vi "Calculate Sample Rate.vi"(0 "data clock rate":dbl=120000000.0 format="%#.3pS/s", 5 "sample rate":dbl=10000000.0 format="%#.3pS/s") -> (4 "decimation sample rate":fxp<+,48,1>, 6 "coerced sample rate":dbl=10000000.0 min=1.0 max=250000000.0 format="%#.3pS/s")   [LabVIEW 2018]
doc: "Calculates the sample rate value to write to the DSP blocks of the device for a requested sample rate, in samples per second."
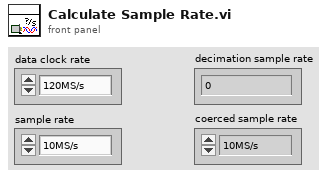
[diagram p1: front panel]
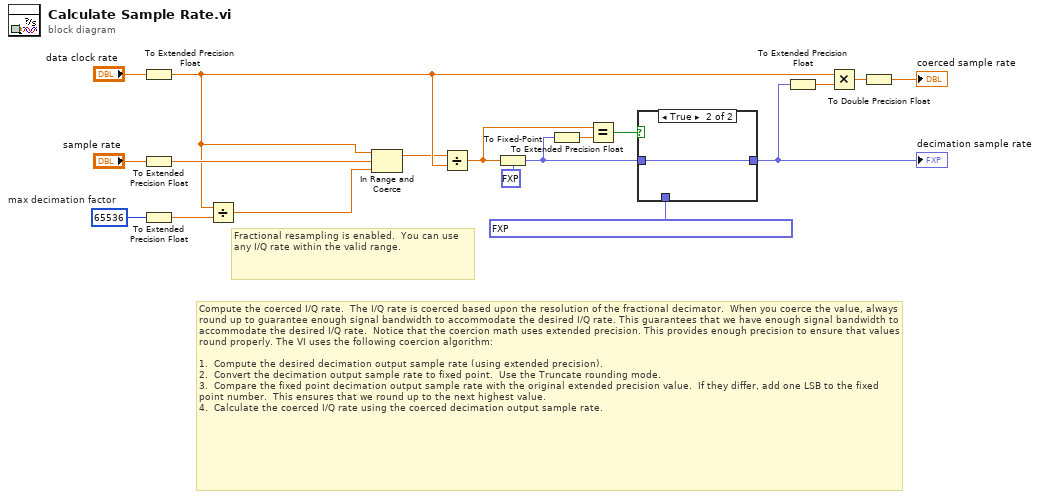
[diagram p0: block diagram]
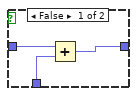
[diagram p2: hidden frame]
diagram:
  w3 = u32 65536  # max decimation factor
  # "Fractional resampling is enabled.  You can use any I/Q rate within the valid range."
  # "Compute the coerced I/Q rate.  The I/Q rate is coerced based upon the resolution of the fractional decimator.  When you coerce the value, always round up to guarantee enough signal bandwidth to accommodate the desired I/Q rate. This guarantees that we have enough signal bandwidth to accommodate the desired I/Q rate.  Notice that the coercion math uses extended precision. This provides enough precision to ensure that values round properly. The VI uses the following coercion algorithm:\n\n1.  Compute the desired decimation output sample rate (using extended precision).\n2.  Convert the decimation output sample rate to fixed point.  Use the Truncate rounding mode.\n3.  Compare the fixed point decimation output sample rate with the original extended precision value.  If they differ, add one LSB to the fixed point number.  This ensures that we round up to the next highest value.\n4.  Calculate the coerced I/Q rate using the coerced decimation output sample rate."
  n1 = To Extended Precision Float(1:"data clock rate") -> (0:w15:ext)
  n2 = To Extended Precision Float(1:"sample rate") -> (0:w18:ext)
  n3 = To Extended Precision Float(1:w3) -> (0:w16:ext)
  n4 = Divide(x=w15, y=w16) -> (x/y=w17:ext)
  n5 = In Range and Coerce(upper limit=w15, x=w18, lower limit=w17) -> (coerced(x)=w9:ext)  [unwired: 1 out]
  n6 = Divide(x=w9, y=w15) -> (x/y=w10:ext)
  n7 = To Fixed-Point(fixed-point type=fxp<+,48,1> 0.0 ("decimation factor"), number=w10) -> (fixed-point=w13:fxp<+,48,1>)
  n8 = To Extended Precision Float(1:w13) -> (0:w11:ext)
  n9 = Equal?(x=w10, y=w11) -> (x = y?=w12:bool)
  n10 = case shown="TRUE" w12 {
    tunnel: w13 -> [w21 w22]
    tunnel: [w19 w22] -> w4
    tunnel: fxp<+,48,1> 7.105427357601002e-15 ("decimation factor") -> [w20 _]
    frame False {
      n11 = Add(x=w21, y=w20) -> (x+y=w19:fxp<+,48,1>)
    }
    frame True {
    }
  }
  "decimation sample rate" <- w4
  n12 = To Extended Precision Float(1:w4) -> (0:w8:ext)
  n13 = Multiply(x=w15, y=w8) -> (x*y=w6:ext)
  n14 = To Double Precision Float(number=w6) -> (double precision float=→"coerced sample rate":dbl)
